vi "Mouse Move.vi"(8 "error in (no error)":errorcluster, 10 "y":i32, 11 "x":i32) -> (0 "error out":errorcluster)   [LabVIEW 2017]
uses:
  <vilib>/Utility/sysdir.llb/System Directory Type.ctl
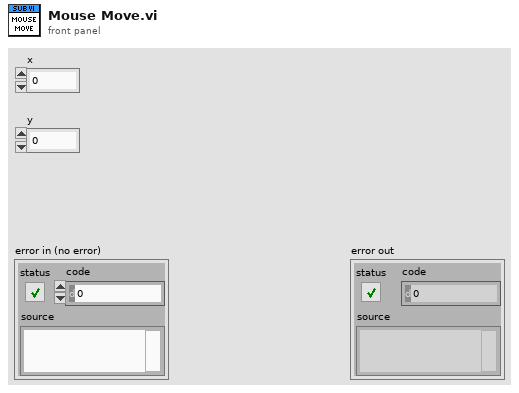
[diagram p1: front panel]
types:
  T1 = typedef "System Directory Type.ctl" = i32
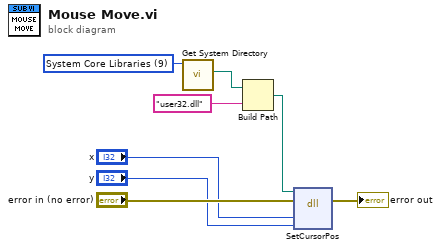
[diagram p0: block diagram]
diagram:
  w6 = T1 9 items=["User Home"=0, "User Desktop"=1, "User Documents"=2, "User Application Data"=3, "User Preferences"=4, "User Temporary"=5, "Public Documents"=6, "Public Application Data"=7, "Public Preferences"=8, "Public Cache"=13, "System Core Libraries"=9, "System Installed Libraries"=10, "Application Files"=11, "Boot Volume Root"=12] ("system directory type")
  n1 = call <vilib>:"Get System Directory.vi"("system directory type"=w6) -> ("system directory"=w5:path)  [unwired: 10 in]
  n2 = Build Path(base path=w5, name or relative path="user32.dll") -> (appended path=w3:path)
  n3 = dll-call lib="C:/Windows/System32/user32.dll" fn="SetCursorPos"(path in=w3, error in="error in (no error)", "x"="x", "y"="y") -> (error out=→"error out":errorcluster)  [unwired: 4 in, 1 out]
